vi "Newton_P(x0) & P'(x0).vi"(10 "x0":dbl, 11 "P(x)":dbl[](array[numeric])) -> (2 "P'(x0)":dbl, 3 "P(x0)":dbl)   [LabVIEW 2018, in "NI_AALPro.lvlib"]
uses:
  <vilib>/Analysis/NI_AALPro.lvlib
  Scalar Polynomial Evaluation (DBL).vi
  nth Derivative of Polynomial (DBL).vi
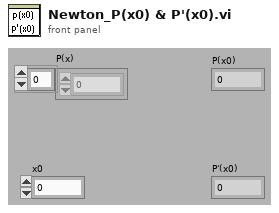
[diagram p1: front panel]
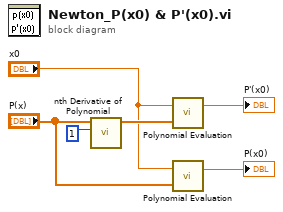
[diagram p0: block diagram]
diagram:
  n1 = call-poly "nth Derivative of Polynomial.vi"("order"=1, "P(x)"="P(x)") -> ("Nth Derivative of P(x)"=w5:dbl[])  [unwired: 8 in, 1 out]
  n2 = call-poly "Polynomial Evaluation.vi"("P(x)"=w5, "a"="x0") -> ("P(a)"=→"P'(x0)":dbl)  [unwired: 1 out]
  n3 = call-poly "Polynomial Evaluation.vi"("P(x)"="P(x)", "a"="x0") -> ("P(a)"=→"P(x0)":dbl)  [unwired: 1 out]
